vi "電流量測值轉換.vi"(10 "input string":string, 11 "Input Data":dbl=222.33) -> (2 "Decimal":i32, 3 "Integer":i32)   [LabVIEW 2019]
uses:
  LLB/Commonly VI/Main Glb.vi
  LLB/Commonly VI.lvlib
panel:
  out "substring":string
  out "F-format string":string
  out "before substring":string
  out "match substring":string
  out "after substring":string
  out "result string":string
  out "number of replacements":i32
  out "offset past replacement":i32
  out "number 2":i32
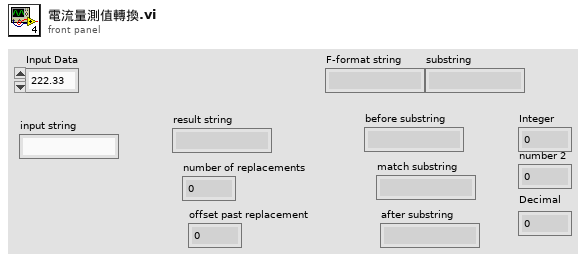
[diagram p1: front panel]
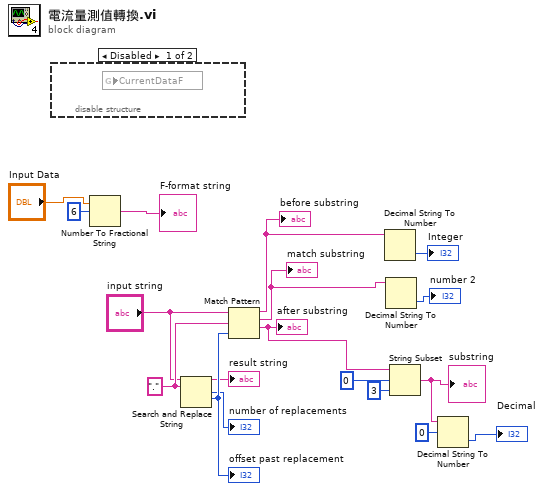
[diagram p0: block diagram]
diagram:
  w11 = "."
  n1 = disable-structure shown="Disabled" {
    frame Disabled {
      n2 = global read "Main Glb.vi" "CurrentDataF"() -> ()  [unwired: 1 in]
    }
    frame Enabled {
    }
  }
  n3 = Number To Fractional String(number="Input Data", width (-)=i16 6) -> (F-format string=→"F-format string":string)  [unwired: 2 in]
  n4 = Search and Replace String(input string="input string", search string=w11) -> (result string=→"result string":string, number of replacements=→"number of replacements":i32, offset past replacement=w14:i32)  [unwired: 6 in, 1 out]
  "offset past replacement" <- w14
  n5 = Match Pattern(string="input string", regular expression=w11, offset (0)=w14) -> (before substring=w15:string, match substring=w16:string, after substring=w6:string)  [unwired: 1 out]
  "before substring" <- w15
  "match substring" <- w16
  "after substring" <- w6
  n6 = Decimal String To Number(string=w15) -> (number=→"Integer":i32)  [unwired: 2 in, 1 out]
  n7 = Decimal String To Number(string=w16) -> (number=→"number 2":i32)  [unwired: 2 in, 1 out]
  n8 = String Subset(string=w6, offset (0)=0, length (rest)=3 ("length (rest)")) -> (substring=w3:string)
  "substring" <- w3
  n9 = Decimal String To Number(string=w3, offset=0) -> (number=→"Decimal":i32)  [unwired: 1 in, 1 out]
